vi "Find Control ref.vi"(8 "error in (no error)":errorcluster caption="错误输入（无错误）", 10 "control name":string="panel0", 11 "panelvi*":refnum<vi>) -> (0 "error out":errorcluster caption="错误输出", 2 "ctrl*":refnum<vi>, 3 "panelvi* out":refnum<vi>)   [LabVIEW 2016]
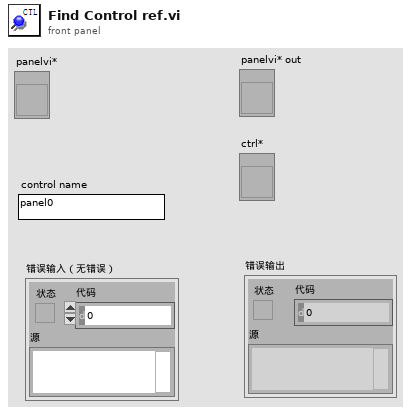
[diagram p1: front panel]
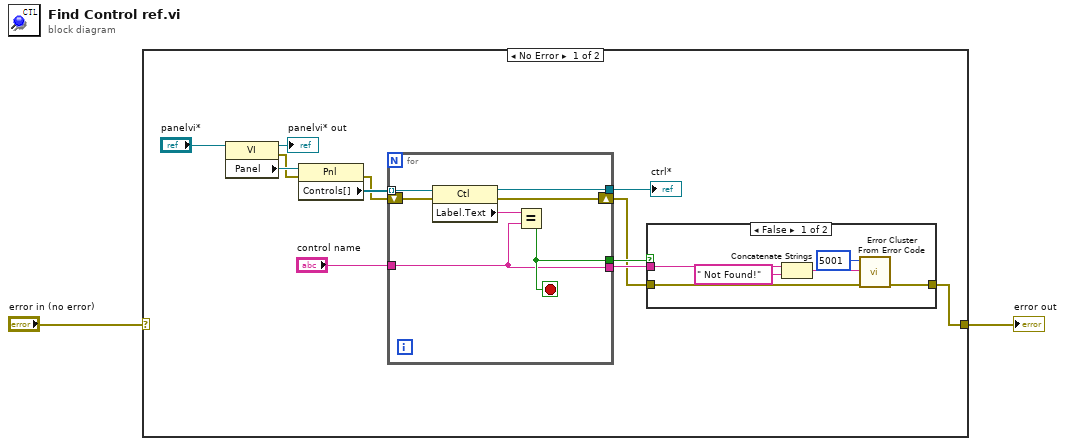
[diagram p0: block diagram]
diagram:
  n1 = case shown="No Error" "error in (no error)" {
    selector: "error in (no error)" -> [_ w29]
    tunnel: [w6 w29] -> w1
    frame No Error {
      n2 = property class="VI"(reference="panelvi*") -> (reference out=→"panelvi* out":refnum<vi>, error out=w8:errorcluster, "Panel"=w14:refnum<vi>)  [unwired: 1 in]
      n3 = property class="Pnl"(reference=w14, error in=w8) -> (error out=w7:errorcluster, "Controls[]"=w11:refnum<vi>[])  [unwired: 1 out]
      n4 = for {
        tunnel: w11 -> [w28] mode=indexing
        tunnel: [w26] -> w13
        tunnel: [w25] -> w9
        tunnel: [w22] -> w10
        shift-right: [w23] -> w5
        shift-left: w7 -> [w24]
        tunnel: "control name" -> [w22]
        stop <- w25 stop-if-true
        n5 = property class="Ctl"(reference=w28, error in=w24) -> (reference out=w26:refnum<vi>, error out=w23:errorcluster, "Label.Text"=w27:string)
        n6 = Equal?(x=w27, y=w22) -> (x = y?=w25:bool)
      }
      "ctrl*" <- w13
      n7 = case shown="False" w9 {
        tunnel: w10 -> [w20 _]
        tunnel: [w16 w21] -> w6
        tunnel: w5 -> [w15 w21]
        frame False {
          n8 = Concatenate Strings(w20, " Not Found!" ("字符串")) -> (w18:string)
          n9 = call <vilib>:"Error Cluster From Error Code.vi"("error in (no error)"=w15, "error message (\"\")"=w18, "error code (0)"=5001) -> ("error out"=w16:errorcluster)  [unwired: 6 in]
        }
        frame True {
        }
      }
    }
    frame Error {
    }
  }
  "error out" <- w1
